vi "题目7.vi"() -> ()   [LabVIEW 2017]
uses:
  <vilib>/Utility/miscctls.llb/LVPositionTypeDef.ctl
  <vilib>/Utility/miscctls.llb/LVBoundsTypeDef.ctl
panel:
  in  "停止":bool
  out "边界":T1
  in  "位置":T2
  in  "闪烁":bool
  in  "键选中":bool
  in  "禁用":T3(ring)
  in  "可见":bool
  in  "数值":dbl
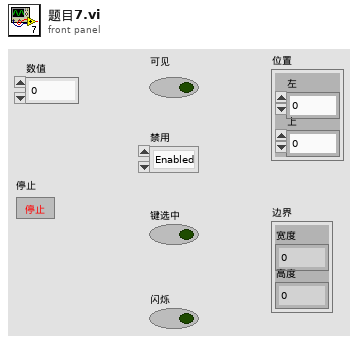
[diagram p1: front panel]
types:
  T1 = typedef "LVBoundsTypeDef.ctl" = cluster{"Width":u32, "Height":u32}
  T2 = typedef "LVPositionTypeDef.ctl" = cluster{"Left":i32, "Top":i32}
  T3 = enum8{"Enabled", "Disabled", "Disabled and Grayed Out"}
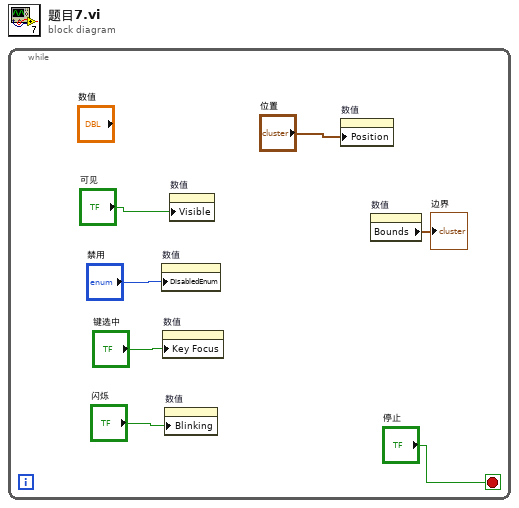
[diagram p0: block diagram]
diagram:
  n1 = while {
    stop <- "停止" stop-if-true
    n2 = property on="数值" class="DigNum (严格)"("DisabledEnum"="禁用") -> ()  [unwired: 2 in, 2 out]
    n3 = property on="数值" class="DigNum (严格)"("Key Focus"="键选中") -> ()  [unwired: 2 in, 2 out]
    n4 = property on="数值" class="DigNum (严格)"("Blinking"="闪烁") -> ()  [unwired: 2 in, 2 out]
    n5 = property on="数值" class="DigNum (严格)"("Visible"="可见") -> ()  [unwired: 2 in, 2 out]
    n6 = property on="数值" class="DigNum (严格)"("Position"="位置") -> ()  [unwired: 2 in, 2 out]
    n7 = property on="数值" class="DigNum (严格)"() -> ("Bounds"=→"边界":T1)  [unwired: 2 in, 2 out]
  }
